vi "Save2.vi"(0 "Save Path":path, 1 "Main folder":string, 2 "DUT":string, 3 "Pass/fail":string, 5 "error in (no error)":errorcluster) -> (14 "Fileout":path, 19 "error out":errorcluster)   [LabVIEW 2024, in "Test_2.lvlib"]
uses:
  Test_2.lvlib
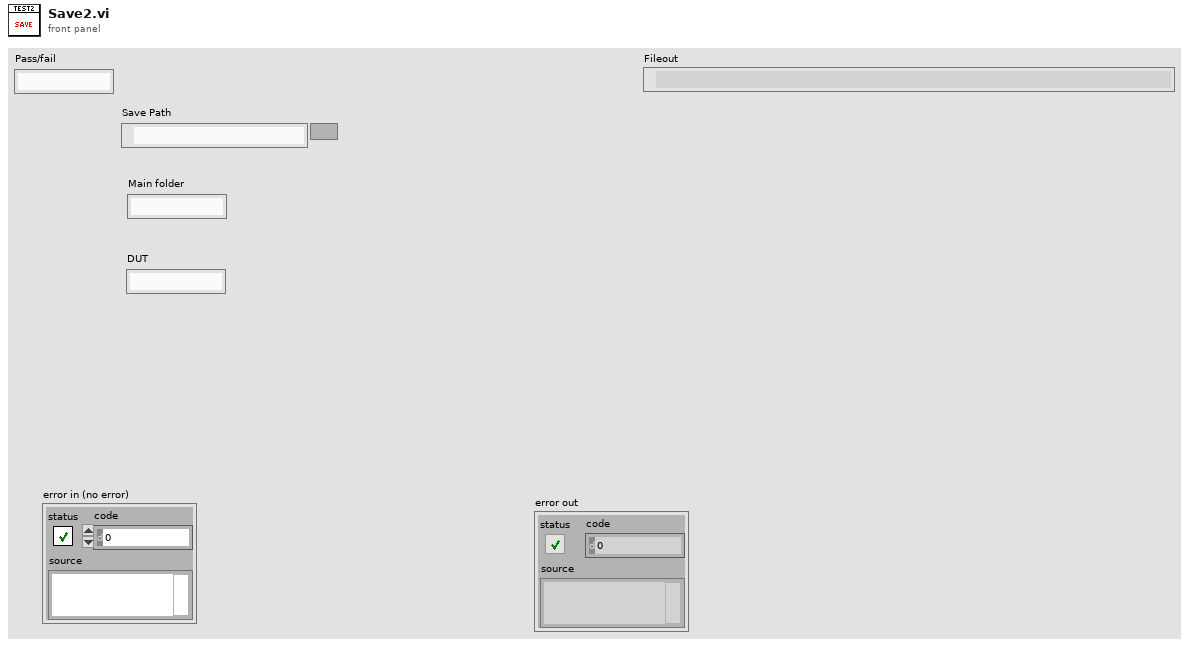
[diagram p1: front panel]
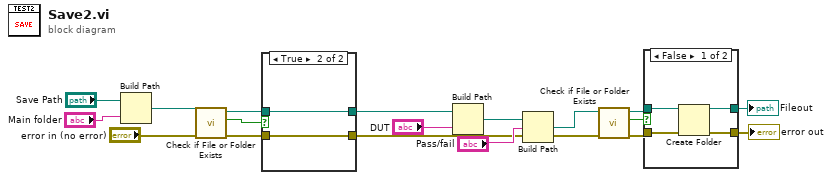
[diagram p0: block diagram]
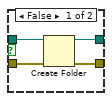
[diagram p3: hidden frame]
diagram:
  n1 = Build Path(base path="Save Path", name or relative path="Main folder") -> (appended path=w16:path)
  n2 = call <vilib>:"Check if File or Folder Exists.vi"("error in (no error)"="error in (no error)", "path"=w16) -> ("error out"=w13:errorcluster, "file or folder exists?"=w14:bool, "dup path"=w12:path)  [unwired: 7 in]
  n3 = case shown="True" w14 {
    tunnel: w13 -> [w22 w23]
    tunnel: w12 -> [w21 w24]
    tunnel: [w20 w23] -> w6
    tunnel: [w19 w24] -> w11
    frame False {
      n4 = Create Folder(path (use dialog)=w21, error in=w22) -> (created path=w19:path, error out=w20:errorcluster)  [unwired: 1 in, 1 out]
    }
    frame True {
    }
  }
  n5 = Build Path(base path=w11, name or relative path="DUT") -> (appended path=w9:path)
  n6 = Build Path(base path=w9, name or relative path="Pass/fail") -> (appended path=w7:path)
  n7 = call <vilib>:"Check if File or Folder Exists.vi"("error in (no error)"=w6, "path"=w7) -> ("error out"=w4:errorcluster, "file or folder exists?"=w5:bool, "dup path"=w3:path)  [unwired: 7 in]
  n8 = case shown="False" w5 {
    tunnel: w4 -> [w28 w29]
    tunnel: w3 -> [w27 w30]
    tunnel: [w26 w29] -> w1
    tunnel: [w25 w30] -> w2
    frame False {
      n9 = Create Folder(path (use dialog)=w27, error in=w28) -> (created path=w25:path, error out=w26:errorcluster)  [unwired: 1 in, 1 out]
    }
    frame True {
    }
  }
  "Fileout" <- w2
  "error out" <- w1
